vi "Control-DIFuel-UserVIRun.vi"(8 "Error In":errorcluster, 11 "DSI Reference":refnum<class "DCM-DSI.lvclass">) -> (0 "Error Out":errorcluster, 3 "DSI Reference":refnum<class "DCM-DSI.lvclass">)   [LabVIEW 2016, in "DSI-RT.lvlib"]
uses:
  DSI-RT.lvlib
  Classes/DCM-DSI/DCM-DSI.lvclass
  <vilib>/addons/Software Calibration Management/xSCM/CalPoint.xnode
  <vilib>/addons/Software Calibration Management/xSCM/FaultPoint.xnode
  <vilib>/addons/Software Calibration Management/xSCM/ni_scm.dll
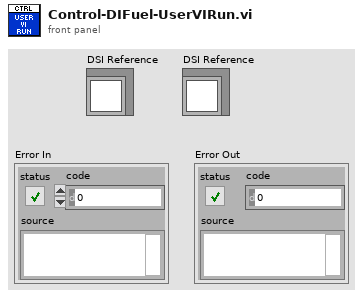
[diagram p1: front panel]
types:
  T1 = typedef "DCM-DSI.lvclass/UserParameter.ctl" = cluster{"Name":string, "Value":dbl}
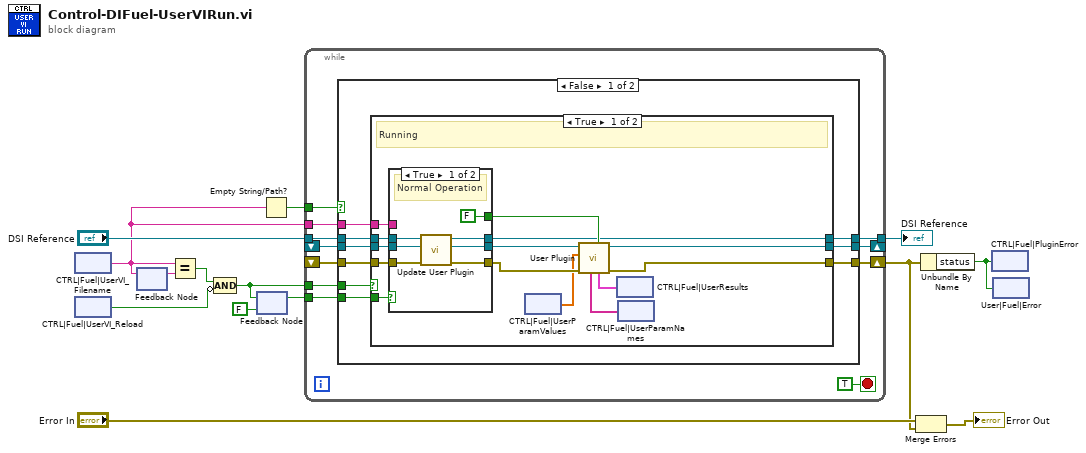
[diagram p0: block diagram]
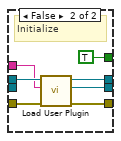
[diagram p2: hidden frame]
diagram:
  n1 = xnode "CTRL|Fuel|UserVI_Filename"() -> ("Value"=w4:string)
  n2 = xnode "CTRL|Fuel|UserVI_Reload"() -> ("Value"=w9:bool)
  n3 = feedback #1() -> (w13:string)  [unwired: 1 in]
  n4 = feedback-in #1(w4) -> ()
  n5 = Equal?(x=w4, y=w13) -> (x = y?=w11:bool)
  n6 = Compound Arithmetic op=AND(w11, invert w9) -> (w12:bool)
  n7 = feedback #2(FALSE) -> (w14:bool)
  n8 = feedback-in #2(w12) -> ()
  n9 = Empty String/Path?(string/path=w4) -> (empty?=w8:bool)
  n10 = while {
    tunnel: w14 -> [w25]
    tunnel: w12 -> [w24]
    tunnel: w4 -> [w23]
    tunnel: w8 -> [w22]
    shift-right: [w18] -> w2
    shift-left: _ -> [w20]
    tunnel: "DSI Reference" -> [w21]
    tunnel: [w19] -> w6
    shift-right: [w16] -> _
    shift-left: _ -> [w15]
    stop <- TRUE stop-if-true
    n11 = case shown="False" w22 {
      tunnel: [w34 w87] -> w19
      tunnel: [w33 _] -> w18
      tunnel: w25 -> [w32 _]
      tunnel: w24 -> [w31 _]
      tunnel: w23 -> [w30 _]
      tunnel: w21 -> [w29 w87]
      tunnel: w20 -> [w28 _]
      tunnel: [w27 _] -> w16
      tunnel: w15 -> [w26 _]
      frame False {
        n12 = case shown="True" w31 {
          tunnel: [w38 w86] -> w34
          tunnel: [w35 _] -> w33
          tunnel: w32 -> [w48 _]
          tunnel: w30 -> [w47 _]
          tunnel: w29 -> [w46 w86]
          tunnel: w28 -> [w45 _]
          tunnel: [w37 _] -> w27
          tunnel: w26 -> [w36 _]
          frame True {
            # "Running"
            n13 = case shown="True" w48 {
              tunnel: [w69 w77] -> w44
              tunnel: [w67 w78] -> w43
              tunnel: w47 -> [_ w74]
              tunnel: w46 -> [w72 w79]
              tunnel: w45 -> [w68 w75]
              tunnel: [FALSE ("Initialize") TRUE ("Initialize")] -> w39
              tunnel: [w70 w76] -> w38
              tunnel: w36 -> [w71 _]
              frame True {
                # "Normal Operation"
                n14 = call "Update User Plugin.vi"("error in (no error)"=w68, "Plugin Reference"=w71, "DSI Reference"=w72) -> ("error out"=w67:errorcluster, "Plugin Reference"=w69:refnum<class "DCM-DSI.lvclass">, "DSI Reference"=w70:refnum<class "DCM-DSI.lvclass">)  [unwired: 6 in]
              }
              frame False {
                # "Initialize"
                n15 = call "Load User Plugin.vi"("error in (no error)"=w75, "Name or relative path"=w74, "DSI Reference"=w79) -> ("error out"=w78:errorcluster, "Plugin Reference"=w77:refnum<class "DCM-DSI.lvclass">, "DSI Reference"=w76:refnum<class "DCM-DSI.lvclass">)  [unwired: 6 in]
              }
            }
            n16 = xnode "CTRL|Fuel|UserParamValues"() -> ("Value"=w40:sgl[])
            n17 = call-dynamic "User Plugin.vi"("Initialize"=w39, "error in (no error)"=w43, "ParamValues"=w40, "DSI Reference"=w44) -> ("error out"=w35:errorcluster, "DSI Reference"=w37:refnum<class "DCM-DSI.lvclass">, "Results"=w41:T1[], "ParamNames"=w42:string[])  [unwired: 4 in]
            n18 = xnode "CTRL|Fuel|UserResults"("Value"=w41) -> ()
            n19 = xnode "CTRL|Fuel|UserParamNames"("Value"=w42) -> ()
          }
          frame False {
            # "Off"
          }
        }
      }
      frame True {
      }
    }
  }
  "DSI Reference" <- w6
  n20 = Merge Errors("Error In", w2) -> (→"Error Out":errorcluster)
  n21 = Unbundle By Name(w2) -> ("status"=w1:bool)
  n22 = xnode "CTRL|Fuel|PluginError"("Value"=w1) -> ()
  n23 = xnode "User|Fuel|Error"("Fault"=w1) -> ()
